vi "WAVE FORM CHART.vi"() -> ()   [LabVIEW 2017]
panel:
  out "Waveform Chart 2":dbl(graph)
  in  "Numeric":dbl format="%#_13g"
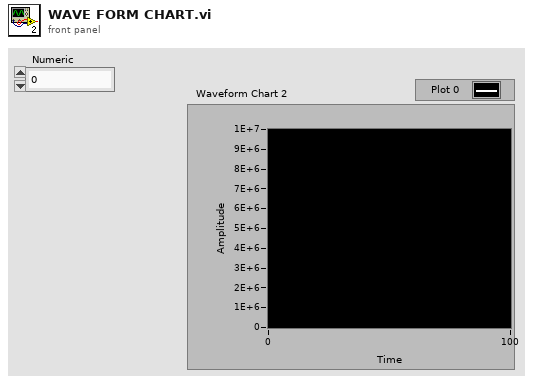
[diagram p1: front panel]
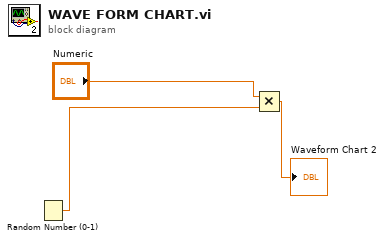
[diagram p0: block diagram]
diagram:
  n1 = Random Number (0-1)() -> (number: 0 to 1=w2:dbl)
  n2 = Multiply(x="Numeric", y=w2) -> (x*y=→"Waveform Chart 2":dbl)
